vi "New NIErrLog Log Provider.vi"(7 "context":string, 8 "error in (no error)":errorcluster, 10 "level":T1 items=["OFF"=0, "FATAL"=100, "ERROR"=200, "WARN"=300, "INFO"=400, "DEBUG"=500, "TRACE"=600, "ALL"=65535]) -> (0 "error out":errorcluster, 3 "Queue Log Provider":refnum<data-value>)   [LabVIEW 2019, in "NIErrLog Log Provider.lvclass"]
doc: "<b>Description</b> Create a new NIErrLog-based logging provider (see Dialog & User Interface Palette / Write to System Log.vi).\n\n<b>Inputs</b>\n<b>context</b>: The default context of the logger. The default context of the logger can be changed using 'Set Context'.\n<b>level</b>: The default logging level of the logger. This level can be chaged using 'Set Log Level'.\n\nBSD 3-Clause License\n\nCopyright (c) 2021, TauTerra, LLC\nAll rights reserved.\n\nRedistribution and use in source and binary forms, with or without\nmodification, are permitted provided that the following conditions are met:\n\n1. Redistributions of source code must retain the above copyright notice, this\n list of conditions and the following disclaimer.\n\n2. Redistributions in binary form must reproduce the above copyright notice,\n this list of conditions and the following disclaimer in the documentation\n and/or other materials provided with the distribution.\n\n3. Neither the name of the copyright holder nor the names of its\n contributors may be used to endorse or promote products derived from\n this software without specific prior written permission.\n\nTHIS SOFTWARE IS PROVIDED BY THE COPYRIGHT HOLDERS AND CONTRIBUTORS \"AS IS\"\nAND ANY EXPRESS OR IMPLIED WARRANTIES, INCLUDING, BUT NOT LIMITED TO, THE\nIMPLIED WARRANTIES OF MERCHANTABILITY AND FITNESS FOR A PARTICULAR PURPOSE ARE\nDISCLAIMED. IN NO EVENT SHALL THE COPYRIGHT HOLDER OR CONTRIBUTORS BE LIABLE\nFOR ANY DIRECT, INDIRECT, INCIDENTAL, SPECIAL, EXEMPLARY, OR CONSEQUENTIAL\nDAMAGES (INCLUDING, BUT NOT LIMITED TO, PROCUREMENT OF SUBSTITUTE GOODS OR\nSERVICES; LOSS OF USE, DATA, OR PROFITS; OR BUSINESS INTERRUPTION) HOWEVER\nCAUSED AND ON ANY THEORY OF LIABILITY, WHETHER IN CONTRACT, STRICT LIABILITY,\nOR TORT (INCLUDING NEGLIGENCE OR OTHERWISE) ARISING IN ANY WAY OUT OF THE USE\nOF THIS SOFTWARE, EVEN IF ADVISED OF THE POSSIBILITY OF SUCH DAMAGE."
uses:
  NIErrLog Log Provider.lvclass
  Log Service/public/level.ctl
  NIErrLog Log Provider.lvclass/NIErrLog Log Provider.ctl
  <vilib>/Utility/SystemLogging/NI_SystemLogging.lvlib
  Log Service/Log Service.lvclass
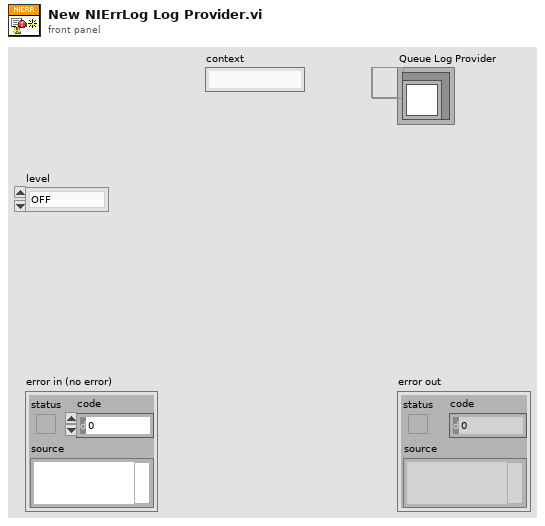
[diagram p1: front panel]
types:
  T1 = typedef "Utility API.lvlib/Log Service.lvclass/level.ctl" = u16
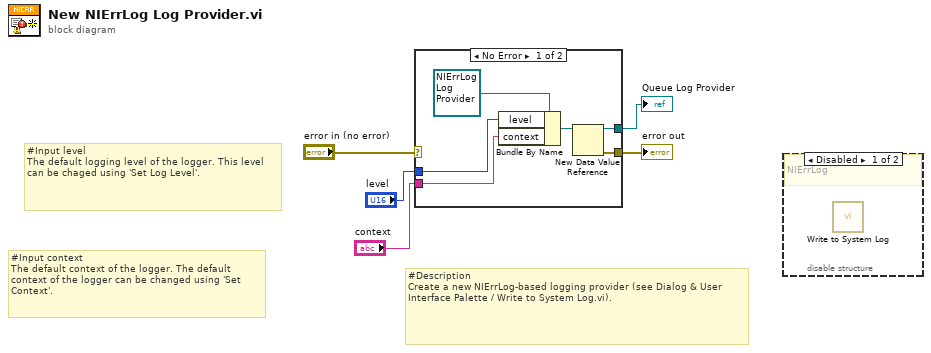
[diagram p0: block diagram]
diagram:
  # "#Input context\nThe default context of the logger. The default context of the logger can be changed using 'Set Context'."
  # "#Input level\nThe default logging level of the logger. This level can be chaged using 'Set Log Level'."
  # "#Description\nCreate a new NIErrLog-based logging provider (see Dialog & User Interface Palette / Write to System Log.vi)."
  n1 = case shown="No Error" "error in (no error)" {
    selector: "error in (no error)" -> [_ w12]
    tunnel: [w9 w12] -> w4
    tunnel: [w7 _] -> w3
    tunnel: "context" -> [w11 _]
    tunnel: "level" -> [w10 _]
    frame No Error {
      n2 = Bundle By Name(cluster=refnum<class "NIErrLog Log Provider.lvclass"> refnum ("Queue Log Provider in"), "level"=w10, "context"=w11) -> (w8:refnum<class "NIErrLog Log Provider.lvclass">)
      n3 = New Data Value Reference(data value=w8) -> (data value reference=w7:refnum<data-value>, error out=w9:errorcluster)  [unwired: 1 in]
    }
    frame Error {
    }
  }
  "error out" <- w4
  "Queue Log Provider" <- w3
  n4 = disable-structure shown="Disabled" {
    frame Disabled {
      # "NIErrLog"
      n5 = call <vilib>:"Write to System Log.vi"() -> ()  [unwired: 11 in, 1 out]
    }
    frame Enabled {
    }
  }
